vi "Stand-Alone Dynamic Signal Analyzer.vi"() -> ()   [LabVIEW 2013]
doc: "Excites a system with a swept sine wave, measures the system's frequency reponse at two points, and calculates the bode plots of the transfer function between those two points in the system.\n\nThis program does this by providing a time while loop in which the Droppable_DSA state machine can run in. \nIn order to include simulated systems, this timed while loop can be replaced with a control and simulation loop. \n\nThis is also where the Droppable_DSA is wired to the corresponding A/D inputs and D/A outputs.\n\n\nInputs:\n\n\n- Excitation Specs:\n\n - Initial Frequency: The lowest frequency of the frequency range which the DSA will measure the bode plot for. \n\n - Final Frequency: The highest frequency of the frequency range which the DSA will measure the bode plot for. \n\n - Frequency Units: Whether the frequecny range input is in Hz or rads/sec. \n \n - Number of Frequencies: The number of logmarithmically spaced frequencies to measure the bode plot for.\n\n - Sampling Time: The time step taking in between each measurement. Also equal to 1/(sampling rate)\n\n - Amplitude: Amplitude of desired swept sine excitation. \n\n - Offset: DC offset of swept sine excitation.\n\n- Cycle Specs:\n\n - Cycles to Settle: The number of cycles of the swept sine wave at each frequency to ignore to let the transcient response die out. \n\n - Cycles to Calculate: The number of cycles of the sept since wave at each frequency to measure in order to measure the bode plot.\n\n- Controls:\n\n - START: Tells the DSA to initalize and then start.\n\n - STOP: Tells the DSA to stop and set all analog outputs to zero.\n\n - EXIT PROGRAM: Tells LabVIEW to set all analog outputs to zero and exit the program.\n\nOutputs:\n\n- Running: Signal to show if the DSA is running.\n\n- Stopped: Signal to show if the DSA is stopped.\n\n- FINISHED LATE: Signal to show if the DSA is running slower than the desired sampling rate. \n\n- Bode Magnitude: The magnitude plot of the TF CH1/CH0.\n\n- Bode Phase: The phase plot of the TF CH1/CH0."
uses:
  <vilib>/Platform/TimedLoop/XDataNode/timing_clust.ctl
  <vilib>/Platform/TimedLoop/XDataNode/nitl_modes.ctl
  <vilib>/Platform/TimedLoop/XDataNode/wakeup.ctl
  <vilib>/myRIO/Instrument Drivers/Onboard IO/AI/vis/Smart Open.vi
  <vilib>/myRIO/Instrument Drivers/Onboard IO/AI/vis/Read.vi
  <vilib>/myRIO/Instrument Drivers/Onboard IO/AO/vis/Smart Open.vi
  <vilib>/myRIO/Instrument Drivers/Onboard IO/AO/vis/Write.vi
  <vilib>/myRIO/Instrument Drivers/Onboard IO/AI/vis/Open.vi
  <vilib>/myRIO/Instrument Drivers/Onboard IO/AO/vis/Open.vi
  <vilib>/myRIO/Common/Instrument Driver Framework/myRIO v1.0/AI/vis/myRIO v1.1 Open AI.vi
  <vilib>/myRIO/Common/Instrument Driver Framework/myRIO v1.0/AO/vis/myRIO v1.1 Open AO.vi
  <vilib>/myRIO/Common/Instrument Driver Framework/Utilities/vis/Validate Channels.vi
  <vilib>/myRIO/Common/Instrument Driver Framework/myRIO v1.0/AI/vis/myRIO v1.0 Reserve AI.vi
  <vilib>/myRIO/Common/Instrument Driver Framework/myRIO v1.0/AO/vis/myRIO v1.0 Reserve AO.vi
  <vilib>/myRIO/Common/Instrument Driver Framework/myRIO v1.0/AI/vis/myRIO v1.0 Build MUX Configuration AI.vi
  <vilib>/myRIO/Common/Instrument Driver Framework/myRIO v1.0/Resource Manager/vis/myRIO v1.0 Reserve Channel List.vi
  <vilib>/myRIO/Common/Instrument Driver Framework/myRIO v1.0/AO/vis/myRIO v1.0 Build MUX Configuration AO.vi
  <vilib>/myRIO/Common/Instrument Driver Framework/myRIO v1.0/Resource Manager/vis/myRIO v1.0 Reserve Channel.vi
  <vilib>/myRIO/Common/Instrument Driver Framework/myRIO v1.0/Resource Manager/vis/myRIO v1.0 Unreserve Channel.vi
  <vilib>/myRIO/Common/Instrument Driver Framework/myRIO v1.0/Resource Manager/vis/myRIO v1.0 Build Mutex Name.vi
  <vilib>/myRIO/Common/Instrument Driver Framework/myRIO v1.0/myRIO v1.1 Open.vi
  <vilib>/myRIO/Common/Instrument Driver Framework/myRIO v1.0/AI/vis/myRIO v1.0 Get Scaling Constants AI.vi
  <vilib>/Utility/VariantDataType/GetNumericInfo.vi
  <vilib>/Utility/error.llb/Error Cluster From Error Code.vi
  <vilib>/myRIO/Common/Instrument Driver Framework/Utilities/vis/IO Manager.vi
  <vilib>/myRIO/Common/Instrument Driver Framework/Utilities/vis/Configuration Manager.vi
  <vilib>/myRIO/Common/Instrument Driver Framework/myRIO v1.0/myRIO v1.0 Close.vi
  <vilib>/myRIO/Common/Instrument Driver Framework/myRIO v1.0/AI/vis/myRIO v1.0 Read AI.vi
  <vilib>/myRIO/Common/Instrument Driver Framework/myRIO v1.0/AO/vis/myRIO v1.0 Get Scaling Constants AO.vi
  <vilib>/myRIO/Common/Instrument Driver Framework/myRIO v1.0/AO/vis/myRIO v1.0 Write AO.vi
  <vilib>/Platform/TimedLoop/XDataNode/XDataNode.xnode
  <vilib>/Platform/TimedLoop/XDataNode/XDNodeRunTimeDep.lvlib
panel:
  in  "Tab Control":T1(tab)
  in  "Excitation Specs":T2={"Initial Frequency"=1.0, "Final Frequency"=1000.0, "Number of Frequencies"=30, "Samping Time [s]"=0.0005, "Amplitude [V]"=1.0, "Offset [V]"=0.0, "Freq Unit"=TRUE}
  in  "Cycle Specs":T3={"Cycles To Settle (M)"=5, "Cycles To Calculate (N)"=5}
  in  "START":bool
  out "Running":bool
  out "Bode Magnitude":cluster{dbl[], dbl[]}(graph)={[1.0, 1.2689610031679222, 1.6102620275609394, 2.043359717856942, 2.592943797404667, 3.2903445623126686, 4.1753189365604015, 5.298316906283708, 6.7233575364993365, 8.531678524172808, 10.826367338740546, 13.73823795883263, 17.43328822199988, 22.122162910704493, 28.072162039411772, 35.62247890262442, 45.20353656360243, 57.36152510448679, 72.7895384398315, 92.36708571873861, 117.21022975334806, 148.73521072935117, 188.73918221350976, 239.5026619987486, 303.9195382313198, 385.6620421163472, 489.3900918477494, 621.0169418915616, 788.0462815669912, 1000.0], [1.0018651131002922, 1.0016050465725763, 1.0010062349698785, 1.0002931137870483, 0.9991459144089636, 0.9972202532472595, 0.9944020144562293, 0.9903082002861369, 0.983855401702225, 0.9738705481650444, 0.9582906977613652, 0.9358034848813956, 0.9036393454169751, 0.857649976648417, 0.7964400088413218, 0.7217565791716765, 0.6359239660806931, 0.5476382842843324, 0.461415834347026, 0.38116988425483045, 0.3091314427820101, 0.2514928062528439, 0.20170891904461263, 0.15879614847289658, 0.127858110424497, 0.10171304349328705, 0.08081117825531599, 0.06376794604720305, 0.050469140870365095, 0.039745706120179934]}
  out "Bode Phase":cluster{dbl[], dbl[]}(graph)={[1.0, 1.2689610031679222, 1.6102620275609394, 2.043359717856942, 2.592943797404667, 3.2903445623126686, 4.1753189365604015, 5.298316906283708, 6.7233575364993365, 8.531678524172808, 10.826367338740546, 13.73823795883263, 17.43328822199988, 22.122162910704493, 28.072162039411772, 35.62247890262442, 45.20353656360243, 57.36152510448679, 72.7895384398315, 92.36708571873861, 117.21022975334806, 148.73521072935117, 188.73918221350976, 239.5026619987486, 303.9195382313198, 385.6620421163472, 489.3900918477494, 621.0169418915616, 788.0462815669912, 1000.0], [-1.4001864556390353, -1.7425257743205063, -2.2774811113746067, -2.940300047591337, -3.797024621582645, -4.874740361894845, -6.244214499985965, -7.9488896703659435, -10.107416371370137, -12.8129960492024, -16.195047872218314, -20.2121008365249, -24.982209581081694, -30.62002310970157, -36.70295501035055, -43.18506539585506, -49.773026506300724, -56.0120451118291, -61.68921924132383, -66.61507141784128, -71.21117465500357, -75.07757805867544, -77.49128997241446, -81.82799122918105, -82.40583459630555, -84.09391534817092, -87.5421411007668, -88.23137376055858, -91.93060722680163, -98.46625820370649]}
  out "FINISHED LATE":bool
  out "Stopped":bool=TRUE
  in  "STOP":bool
  out "Live Signals":cluster{"DSA Excitation":dbl, "output y(t)":dbl}(graph)={"DSA Excitation"=0.004882813, "output y(t)"=-0.009765626}
  in  "Exist Porgram":bool
  # "PMCL Dynamic Signal Analyzer"
  # "Magnitude"
  # "Magnitude"
  # "Dynamic Signal Analyzer"
  # "Controls"
  # "Operation"
  # "Wiring"
  # "AO 0:   System Reference\n \nAI   0:   TF Input\n \nAI   1:   TF Output"
  # "Phase"
  # "Phase"
  # "Excitation Frequencies"
  # "Frequency\nUnits"
  # "[Hz]"
  # "Excitation Magnitude"
  # "[rad/s]"
  # "Running the DSA"
  # "Collecting Data\n \n(1) Right click the graph and select Export.\n \n      - NOTE: You can only record what is shown on the graph!\n\n(2) Choose the format you want to export your data to.\n \n       - Export Data To Clipboard: Copies it so you can paste it into a program like Matlab\n \n       - Export Data To Excel: Opens up your data in Excel.\n \n       - Export Simpliefed Image... : Saves your data as a cleaned up screenshot picture\n  \n Changing What You Record\n \nTo change the length of time displayed on the graph and thus the length of time you record data for, right click and select Chart History Length while the porgram is NOT running. \n \n        Chart History Length = (Desired Length of Time in Sec) / (Controller Sampling Time)"
  # "(1) Press the white arrow above,          , to start the program.\n\n(2) Set the DSA Sampling Time, the rate at which the myRIO collects data and updates the \n      disturbance sent to the plant.\n \n       - Note:   Sampling Rate = 1/(DSA Sampling Time)     where the default is 0.0005 sec which \n                                                                                                              is a sampling rate of 2.0 kHz.\n \n      - Note: If the FINISHED LATE button flashes, the myRIO needs to sample at a slower rate.\n \n(3) Set other desired parameters: \n\n      - Inital Frequency: Atleast 1 decade before frequency of interest\n\n      - Final Frequency: Atleast 1 decade before frequency of interest\n \n             ~ Note:  Max Final Frequency = Sampling Rate/2  where for this case would be 1.25 kHz.          \n\n      - Number of Frequnecies: 30\n\n      - Amplitude: Largest Amplitude such that the control effort does not staturate\n\n      - Cycles to Settle: 5 minimum for low frequencies & 20 minimum for high frequencies\n\n      - Cycles to Calculate: 5 minimum for low frequencies & 20 minimum for high frequencies  \n\n(4) Press START to start the DSA.\n\n(5) Press STOP to stop the DSA if needed or it will stop when it is finished. \n\n(6)  Click EXIT PROGRAM in the upper right hand corner to stop the progam."
  # "Detailed Wiring\n \n(0) General:\n \n       - AO 0: System Reference\n \n       - AI   0- : AGND (Analog Ground)\n \n       - AI   1- : AGND (Analog Ground)\n\n(1) Plant Transfer Function:\n \n \n       - AI   0+: Control Effort (Plant Input)\n \n       - AI   1+: Plant Output (Sensor Ouput if Plant Output is not a voltage)\n\n(2) Return Ratio Transfer Function:\n \n \n       - AI   0+: Error\n \n       - AI   1+:Feedback Output (Sensor Output)\n\n(3) Closed Loop Transfer Function\n \n \n       - AI   0+: System Refence\n \n       - AI   1+: Plant Output  (Sensor Ouput if Plant Output is not a voltage)\n\nNOTE: If AI  1+ is the sensor output instead of the plant output in case (1) & (3), the desired \n             frequency reponses will be gained by the gain of the sensor."
  # "A DSA, or Dynamic Signal Analyzer is a tool that measures a the frequency response of a transfer function and plots its corresponding bode plots."
  # "A DSA works in 3 steps:\n\n      (1) It inputs a swept sine wave (a sine wave that increaes in frequency), D, at the feedback summing junction. This sine wave will show up through out the system with varying magnitudes and phase. It is how \n            the magnidute and phase of this swept sine wave changes is what we care about.\n\n      (2) It measures the signal at two points through out the system.\n\n      (3) It finds the frequency response of the  transfer function between the two points measured. This is easily shown as a bode plot as  the  magnidute of the frequency response is the magnitude of the signal \n           measured at one point divided the  magnitude of the singal at the other point and the phase of the frequency response is the phase of the signal measured at the first point minus the phase of the signal \n           measured at the second point.\n\n\nThe easiest way to explain this is to show how the DSA calculates the frequnecy response for a transfer function is to look how it does it for the 3 transfer functions we care about (plant, return ratio, and closed loop).\n\n      - Plant: The plant TF is just the ratio of the output of the plant to its input. Thus the DSA finds the frequency response of the plant TF by measuring the signal output by the plant (a swept sine wave), Y, and the \n                    signal input to the plant (a swept sine wave), C. Then it divides the magnitude of Y by the magnitude of C and subtracts the phase of C from the phase of Y at each frequency of the swept sine wave. This \n                     provides the frequency reponse of the plant as it changes with freqency.\n\n      - Return Ratio: The return ratio TF is just the ratio of the output of the loop to its input. Thus the DSA finds the frequency response of the return ratio TF by measuring the signal output by the loop (a swept sine \n                                 wave), M, and the signal input to the loop (a swept sine wave), E. Then it divides the magnitude of M by the magnitude of E and subtracts the phase of E from the phase of M at each frequency of \n                                 the swept sine wave. This provides the frequency reponse of the plant as it changes with freqency.\n\n      - Closed Loop: The closed loop TF is just the ratio of the output of the closed loop to its input. Thus the DSA finds the frequency response of the closed loop TF by measuring the signal output by the closed loop \n                                 (a swept sine  wave), Y, and the signal input to the closed loop (a swept sine wave), R. Then it divides the magnitude of Y by the magnitude of R and subtracts the phase of R from the phase of Y at \n                                  each frequency of the swept sine wave. This provides the frequency reponse of the plant as it changes with freqency."
  # "Copyright (c) 2015 Tyler Hamer\n\nPermission is hereby granted, free of charge, to any person obtaining a copy of this software and associated documentation files (the \"Software\"), to deal in the Software without restriction, including without limitation the rights to use, copy, modify, merge, publish, and/or distribute, but not sublicense, and/or sell copies of the Software, and to permit persons to whom the Software is furnished to do so, subject to the following conditions:\n\nThe above copyright notice and this permission notice shall be included in all copies or substantial portions of the Software.\n\nTHE SOFTWARE IS PROVIDED \"AS IS\", WITHOUT WARRANTY OF ANY KIND, EXPRESS OR IMPLIED, INCLUDING BUT NOT LIMITED TO THE WARRANTIES OF MERCHANTABILITY, FITNESS FOR A PARTICULAR PURPOSE AND NONINFRINGEMENT. IN NO EVENT SHALL THE AUTHORS OR COPYRIGHT HOLDERS BE LIABLE FOR ANY CLAIM, DAMAGES OR OTHER LIABILITY, WHETHER IN AN ACTION OF CONTRACT, TORT OR OTHERWISE, ARISING FROM, OUT OF OR IN CONNECTION WITH THE SOFTWARE OR THE USE OR OTHER DEALINGS IN THE SOFTWARE"
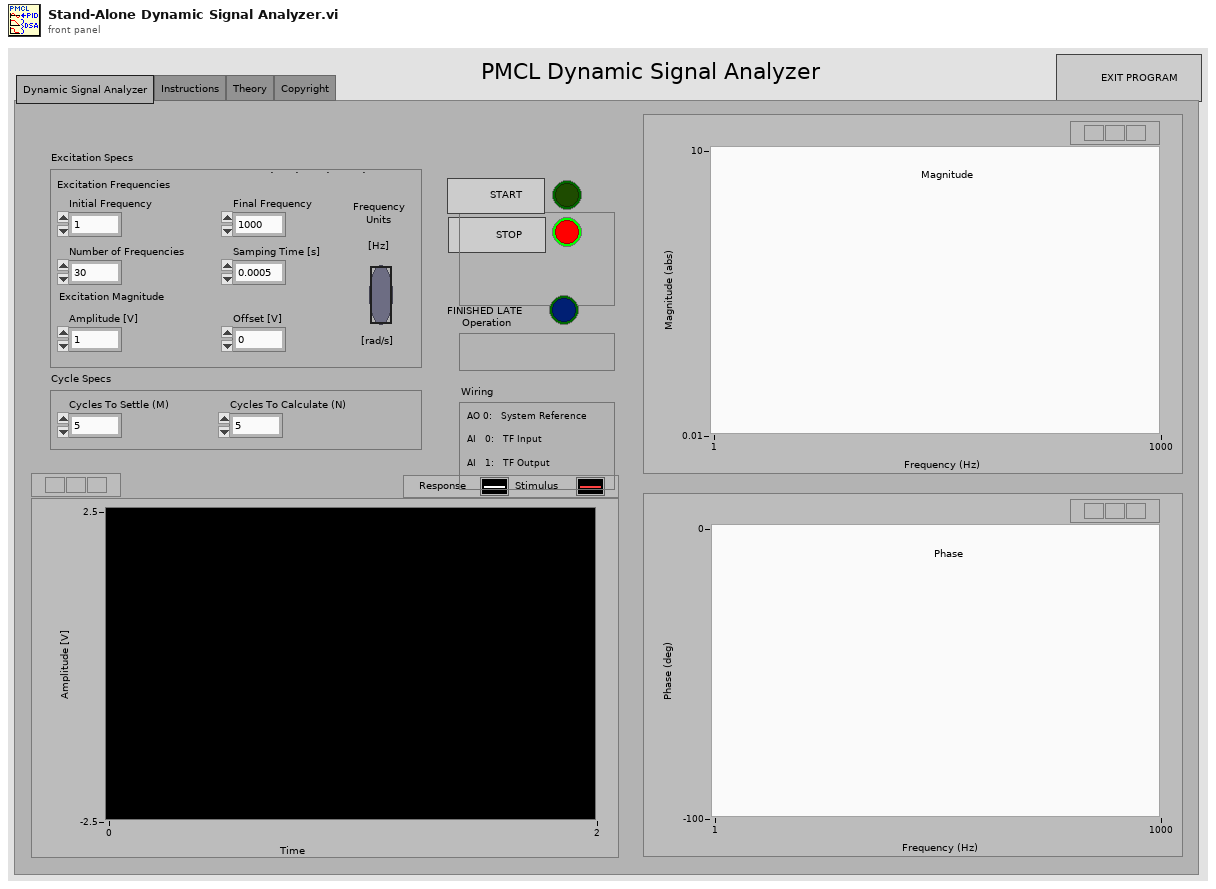
[diagram p1: front panel]
types:
  T1 = enum32{"Dynamic Signal Analyzer", "Instructions", "Theory", "Copyright"}
  T2 = cluster{"Initial Frequency":dbl, "Final Frequency":dbl, "Number of Frequencies":i16, "Samping Time [s]":dbl, "Amplitude [V]":dbl, "Offset [V]":dbl, "Freq Unit":bool}
  T3 = cluster{"Cycles To Settle (M)":i16, "Cycles To Calculate (N)":i16}
  T4 = typedef "XDNodeRunTimeDep.lvlib/timing_clust.ctl" = cluster{"Expected End [f-1]":u64, "Actual End [f-1]":u64, "Finished Late? [f-1]":bool, "Expected End [i-1]":u64, "Actual End [i-1]":u64, "Finished Late? [i-1]":bool, "Expected Start [i]":u64, "Actual Start [i]":u64, "Expected Start [f]":u64, "Actual Start [f]":u64, "Source Name":string, "Structure Name":string, "Period":i64, "Deadline":i64, "Offset":i64, "Start":i64, "Priority":i32, "Timeout":i32, "Mode":T5, "Wakeup Reason":T6, "Error":errorcluster, "Source Type":string, "Secondary Source Type":string, "Global End Time":u64, "Global Start Time":u64, "Frame Duration":u64, "Iteration Duration":u64, "Assigned CPU":i32, "I/O Scan Engine Mode":u32}
  T5 = typedef "XDNodeRunTimeDep.lvlib/nitl_modes.ctl" = enum32{"No Change", "Process missed periods, maintain original phase", "Discard missed periods, maintain original phase", "Process missed periods, ignore original phase", "Discard missed periods, ignore original phase"}
  T6 = typedef "XDNodeRunTimeDep.lvlib/wakeup.ctl" = enum32{"Normal", "Aborted", "Asynchronous wakeup", "Timing source error", "Timed loop error", "Timeout"}
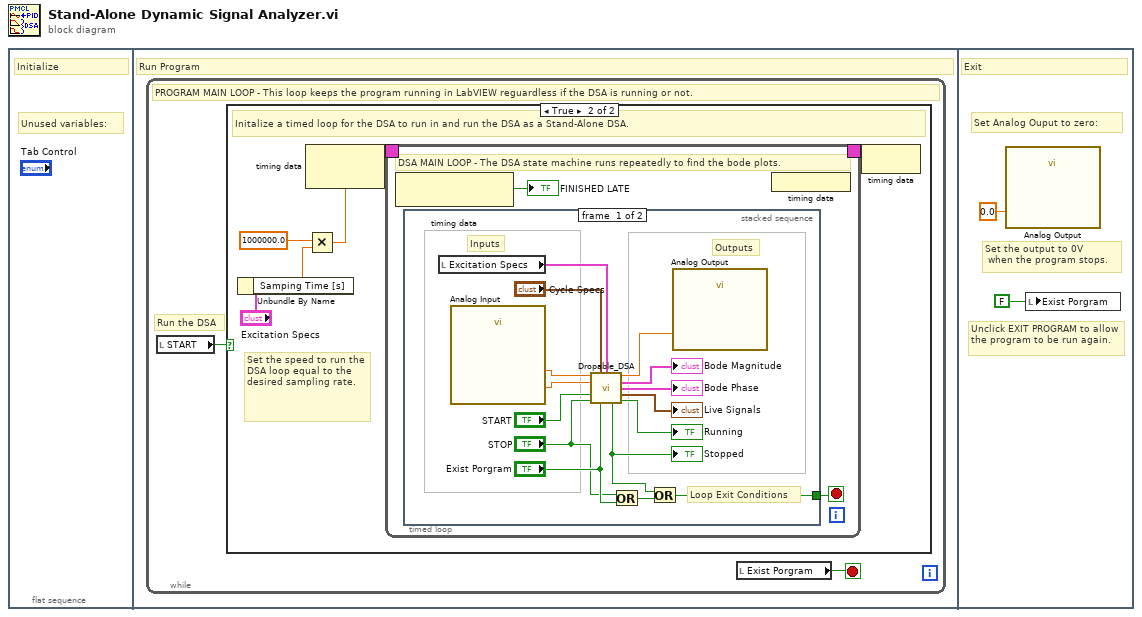
[diagram p0: block diagram]
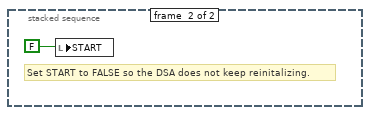
[diagram p3: hidden frame]
diagram:
  n1 = flat-sequence {
    frame #0 {
      # "Unused variables:"
      # "Initialize"
    }
    frame #1 {
      # "Run Program"
      n2 = while {
        stop <- w2 stop-if-true
        # "Run the DSA"
        # "PROGRAM MAIN LOOP - This loop keeps the program running in LabVIEW reguardless if the DSA is running or not."
        n3 = local read "START"() -> (w1:bool)
        n4 = case shown="True" w1 {
          frame False {
            # "FALSE = Do Nothing"
          }
          frame True {
            # "Set the speed to run the DSA loop equal to the desired sampling rate."
            # "Initalize a timed loop for the DSA to run in and run the DSA as a Stand-Alone DSA."
            n5 = Unbundle By Name("Excitation Specs") -> ("Samping Time [s]"=w5:dbl)
            n6 = Multiply(x=1000000.0, y=w5) -> (x*y=w3:dbl)
            n7 = node-c288(w3) -> (w8:T4)
            n8 = timed-loop {
              timing: w8 -> [_]
              timing-out: [_] -> w7
              stop <- w9 stop-if-true
              # "DSA MAIN LOOP - The DSA state machine runs repeatedly to find the bode plots."
              n9 = node-c288() -> (→"FINISHED LATE":bool)  [unwired: 1 in]
              n10 = stacked-sequence {
                tunnel: [w11 _] -> w9
                frame #0 {
                  # "Loop Exit Conditions"
                  # "Outputs"
                  # "Inputs"
                  n11 = local read "Excitation Specs"() -> (w18:T2)
                  n12 = call "Analog Input"() -> ("System Output (C/AI1)"=w16:dbl, "System Input (C/AI0)"=w17:dbl)  [unwired: 25 in, 1 out]
                  n13 = call "Dropable_DSA.vi"("Analog In CH1"=w16, "Cycle Specs"="Cycle Specs", "Excitation Specs"=w18, "Analog In CH0"=w17, "START"="START", "STOP"="STOP", "Exist Porgram"="Exist Porgram") -> ("Analog Out"=w22:dbl, "Bode Magnitude"=→"Bode Magnitude":cluster{dbl[], dbl[]}, "Bode Phase"=→"Bode Phase":cluster{dbl[], dbl[]}, "Live Signals"=→"Live Signals":cluster{"DSA Excitation":dbl, "output y(t)":dbl}, "Stopped"=w12:bool, "Running"=→"Running":bool)  [unwired: 3 in]
                  "Stopped" <- w12
                  n14 = Or(x="STOP", y="Exist Porgram") -> (x .or. y?=w13:bool)
                  n15 = Or(x=w12, y=w13) -> (x .or. y?=w11:bool)
                  n16 = call "Analog Output"("System Input (C/AO0)"=w22) -> ()  [unwired: 26 in, 1 out]
                }
                frame #1 {
                  # "Set START to FALSE so the DSA does not keep reinitalizing."
                  n17 = local write "START"(FALSE) -> ()
                }
              }
              n18 = node-c288() -> ()  [unwired: 1 out]
            }
            n19 = node-c288(w7) -> ()
          }
        }
        n20 = local read "Exist Porgram"() -> (w2:bool)
      }
    }
    frame #2 {
      # "Unclick EXIT PROGRAM to allow the program to be run again."
      # "Set Analog Ouput to zero:"
      # "Set the output to 0V\n when the program stops."
      # "Exit"
      n21 = call "Analog Output"("System Input (C/AO0)"=0.0 ("C/AO1")) -> ()  [unwired: 26 in, 1 out]
      n22 = local write "Exist Porgram"(FALSE) -> ()
    }
  }
